vi "TCP_Cli.vi"() -> ()   [LabVIEW 2016]
panel:
  in  "立显/保存":bool
  in  "显示字符":string="立即显示美丽洛阳"
  in  "发送":bool
  in  "停止":bool
  out "接收到得原始数据":string
  in  "输入端口号":u64=10001
  in  "输入连接IP":string="192.168.1.200"
  # "FFFF FFFF FFFF 0000 0000 7834 0100 2100 0000 0000 0000 0000 00A0 D4A5"
  # "开机"
  # "FFFF FFFF FFFF 0000 0000 7834 0100 2200 0000 0000 0000 0000 00AF 90A5"
  # "关机"
  # "5A48 0738 740B 0000 0000 7934 0100 2944 9100 0000 0000 0000 0000 003F 89A5"
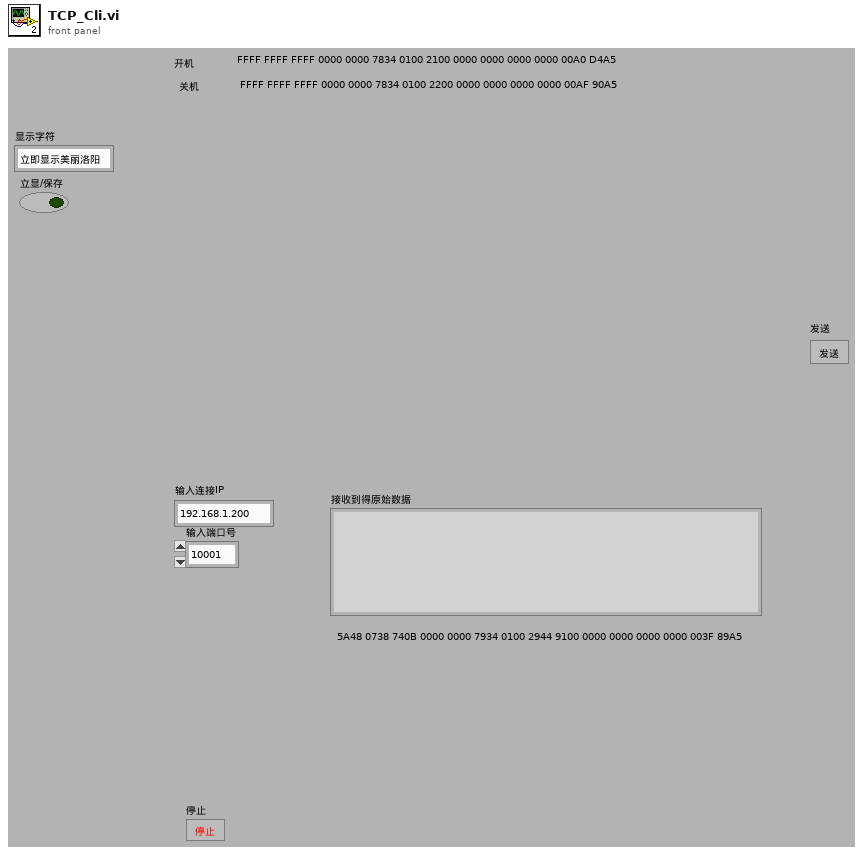
[diagram p1: front panel]
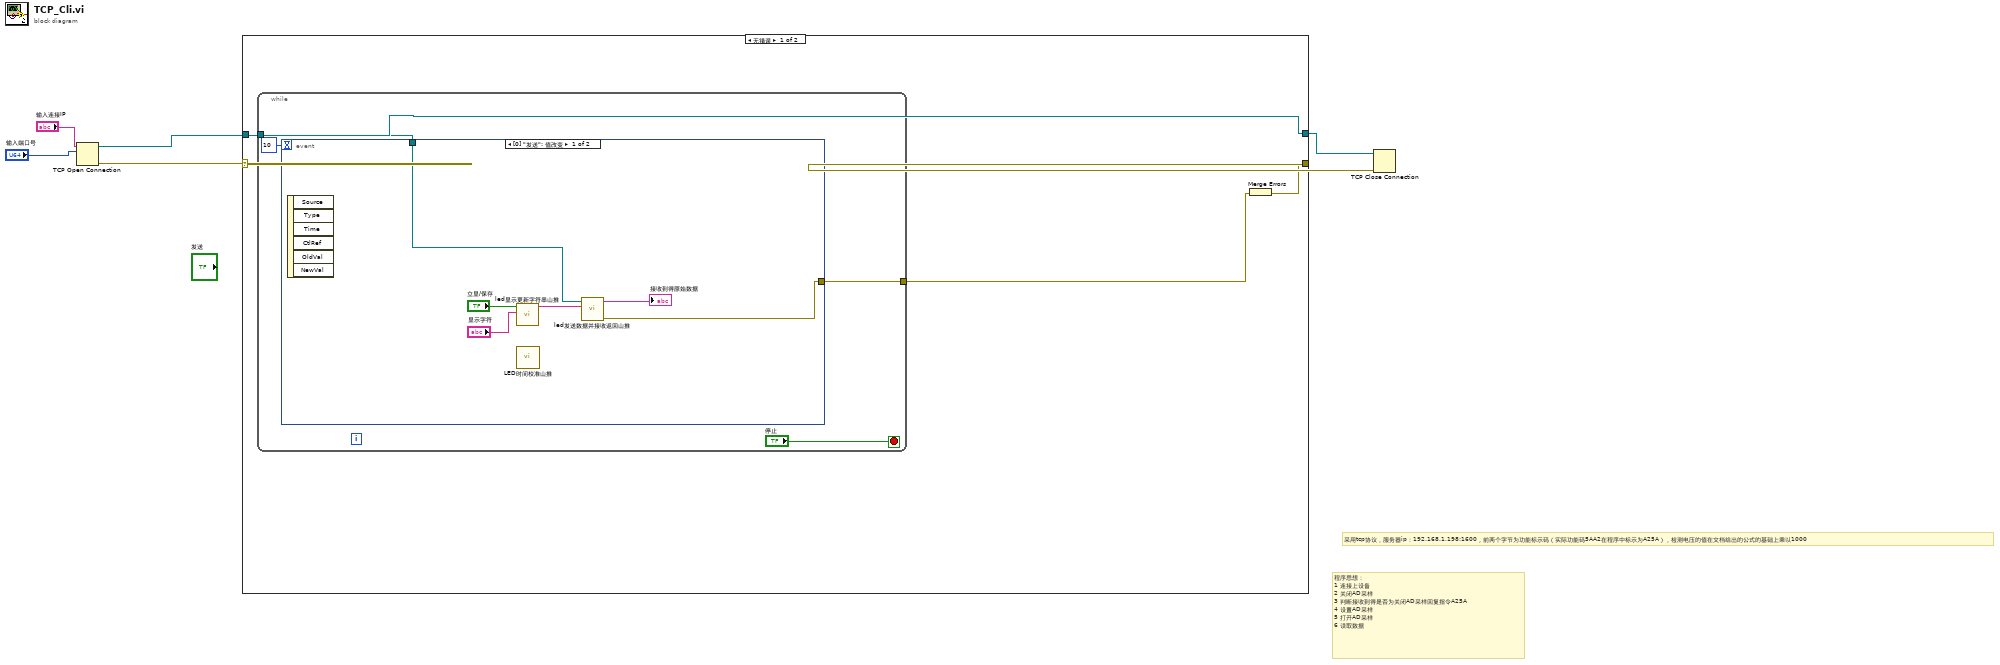
[diagram p0: block diagram]
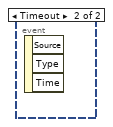
[diagram p2: hidden frame]
diagram:
  # "程序思想：\n1 连接上设备\n2 关闭AD采样\n3 判断接收到得是否为关闭AD采样回复指令A25A\n4 设置AD采样\n5 打开AD采样\n6 读取数据"
  # "采用tcp协议，服务器ip：192.168.1.198:1600，前两个字节为功能标示码（实际功能码5AA2在程序中标示为A25A），检测电压的值在文档给出的公式的基础上乘以1000"
  n1 = TCP Open Connection(address="输入连接IP", remote port or service name="输入端口号") -> (connection ID=w5:refnum<k5>, error out=w4:errorcluster)  [unwired: 3 in]
  n2 = case shown="无错误" w4 {
    selector: w4 -> [_ w21]
    tunnel: w5 -> [w7 w20]
    tunnel: [w9 w21] -> w3
    tunnel: [w7 w20] -> w2
    frame No Error {
      n3 = while {
        tunnel: [w13] -> w8
        tunnel: w7 -> [w12]
        stop <- "停止" stop-if-true
        n4 = event shown="[0] \"发送\": 值改变" {
          selector: _ -> [_ _]
          dyn-events: _ -> [_ _]
          timeout: 10 -> [_ _]
          tunnel: [w15 _] -> w13
          tunnel: w12 -> [w14 _]
          event "发送": Value Change {
            n5 = event-data() -> ()  [unwired: 1 in, 6 out]
            n6 = call "led显示更新字符串山推.vi"("显示字符"="显示字符", "立显/保存"="立显/保存") -> ("发送数据"=w17:string)  [unwired: 9 in]
            n7 = call "LED时间校准山推.vi"() -> ()  [unwired: 11 in, 1 out]
            n8 = call "led发送数据并接收返回山推.vi"("发送数据"=w17, "TCP网络连接输入"=w14) -> ("错误输出"=w15:errorcluster, "接收到得原始数据"=→"接收到得原始数据":string)  [unwired: 8 in]
          }
          event Timeout {
            n9 = event-data() -> ()  [unwired: 1 in, 3 out]
          }
        }
      }
      n10 = Merge Errors(w8) -> (w9:errorcluster)
    }
    frame Error {
    }
  }
  n11 = TCP Close Connection(connection ID=w2, error in (no error)=w3) -> ()  [unwired: 1 in, 2 out]
